vi "Area.vi"(11 "Circle in":T1) -> (2 "Area":dbl, 3 "Circle Out":T1)   [LabVIEW 2015, in "Circle Library.lvlib"]
uses:
  Circle Library.lvlib
  Circle cluster.ctl
  colors.ctl
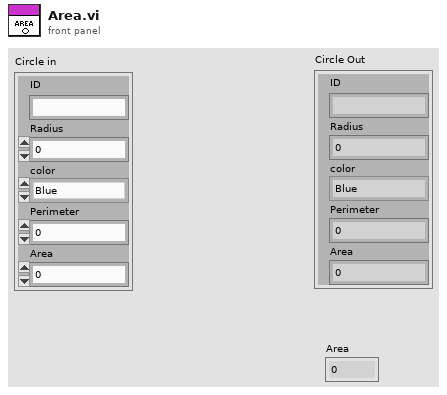
[diagram p1: front panel]
types:
  T1 = typedef "Circle Library.lvlib/Circle cluster.ctl" = cluster{"ID":string, "Radius":dbl, "color":T2, "Perimeter":dbl, "Area":dbl}
  T2 = typedef "colors.ctl" = enum16{"Blue", "Red", "Green", "Yellow"}
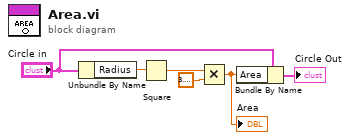
[diagram p0: block diagram]
diagram:
  n1 = Unbundle By Name("Circle in") -> ("Radius"=w6:dbl)
  n2 = Square(x=w6) -> (x^2=w5:dbl)
  n3 = Multiply(x=w5, y=3.141592653589793) -> (x*y=w1:dbl)
  "Area" <- w1
  n4 = Bundle By Name(cluster="Circle in", "Area"=w1) -> (→"Circle Out":T1)
